vi "Client_Post.vi"() -> ()   [LabVIEW 2020]
uses:
  <vilib>/httpClient/POSTBuffer.vi
  <vilib>/httpClient/LabVIEWHTTPClient.lvlib
panel:
  out "body":string
  out "headers":string
  # "{\"Nom\":\"\",\"Age\":0}"
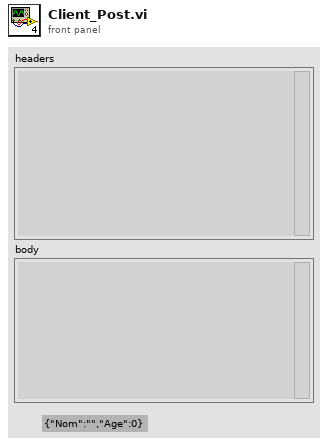
[diagram p1: front panel]
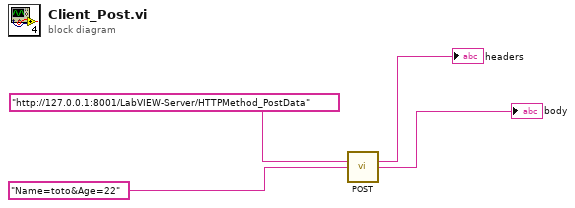
[diagram p0: block diagram]
diagram:
  n1 = call-poly <vilib>:"POST.vi"("url"="http://127.0.0.1:8001/LabVIEW-Server/HTTPMethod_PostData", "buffer"="Name=toto&Age=22") -> ("headers"=→"headers":string, "body"=→"body":string)  [unwired: 10 in, 2 out]
